vi "Run.vi"() -> ()   [LabVIEW 2016, in "TestLibrary.lvlib"]
uses:
  TestLibrary.lvlib
  <vilib>/SLL Drona/Drona.lvlib
panel:
  out "error out":errorcluster
  in  "error in":errorcluster
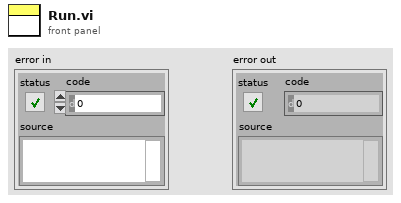
[diagram p1: front panel]
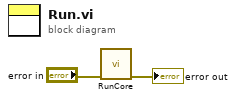
[diagram p0: block diagram]
diagram:
  n1 = call <vilib>:"RunCore.vi"("error in (no error)"="error in") -> ("error out"=→"error out":errorcluster)  [unwired: 10 in]
